vi "Read channels.vi"(8 "error in (no error)":errorcluster, 11 "Numeric Limit Compare Config in":refnum<class "Numeric Limit Compare Config.lvclass">) -> (0 "error out":errorcluster, 2 "Channels":refnum<class "TBM channel.lvclass">[](array[class]), 3 "Numeric Limit Compare Config out":refnum<class "Numeric Limit Compare Config.lvclass">)   [LabVIEW 2015, in "Numeric Limit Compare Config.lvclass"]
uses:
  Numeric Limit Compare Config.lvclass
  <vilib>/NI/Tag Bus Module Framework/channel/TBM channel.lvclass
  Numeric Limit Compare Config.lvclass/Numeric Limit Compare Config.ctl
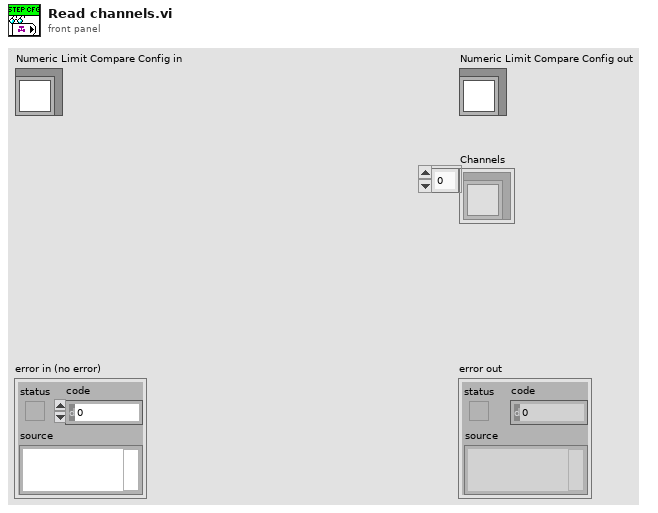
[diagram p1: front panel]
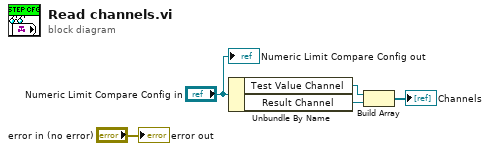
[diagram p0: block diagram]
diagram:
  n1 = Unbundle By Name("Numeric Limit Compare Config in") -> ("Test Value Channel"=w3:refnum<class "TBM channel.lvclass">, "Result Channel"=w2:refnum<class "TBM channel.lvclass">)
  n2 = Build Array(w3, w2) -> (→"Channels":refnum<class "TBM channel.lvclass">[])
  "error out" <- "error in (no error)"
  "Numeric Limit Compare Config out" <- "Numeric Limit Compare Config in"
